vi "ATS_Create_String.vi"(8 "Scale":string="MS/s", 9 "Step":i32=1, 10 "End":i32, 11 "Start":i32) -> (1 "Count":u32, 3 "Range_Out":string[](array[string]))   [LabVIEW 2014]
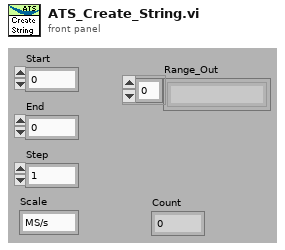
[diagram p1: front panel]
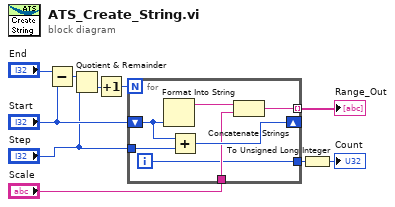
[diagram p0: block diagram]
diagram:
  n1 = Subtract(x="End", y="Start") -> (x-y=w8:i32)
  n2 = Quotient & Remainder(x=w8, y="Step") -> (floor(x/y)=w5:i32)  [unwired: 1 out]
  n3 = Increment(x=w5) -> (x+1=w3:i32)
  n4 = for {
    N: w3 -> [_]
    shift-right: [w13] -> _
    shift-left: "Start" -> [w15]
    tunnel: [w16] -> w6 mode=indexing
    tunnel: "Step" -> [w14]
    tunnel: "Scale" -> [w12]
    tunnel: [w11] -> w2
    i -> [w11]
    n5 = Format Into String(w15) -> (resulting string=w17:string)  [unwired: 3 in, 1 out]
    n6 = Add(x=w15, y=w14) -> (x+y=w13:i32)
    n7 = Concatenate Strings(w17, w12) -> (w16:string)
  }
  "Range_Out" <- w6
  n8 = To Unsigned Long Integer(number=w2) -> (unsigned 32bit integer=→"Count":u32)
